vi "writeToXML.vi"(8 "error in (no error)":errorcluster, 10 "ClassLabel":string, 11 "CommandsForRotatorAxis in":refnum<class "CommandsForRotatorAxis.lvclass">) -> (0 "error out":errorcluster, 2 "XMLout":string, 3 "CommandsForRotatorAxis out":refnum<class "CommandsForRotatorAxis.lvclass">)   [LabVIEW 2014, in "TCSDataDefinitions.lvlib" / "TCSMountControlCommand.lvlib" / "CommandsForRotatorAxis.lvlib" / "CommandsForRotatorAxis.lvclass"]
uses:
  CommandsForRotatorAxis.lvclass
  TCSMCCCommand/TCSMCCCommand.lvclass
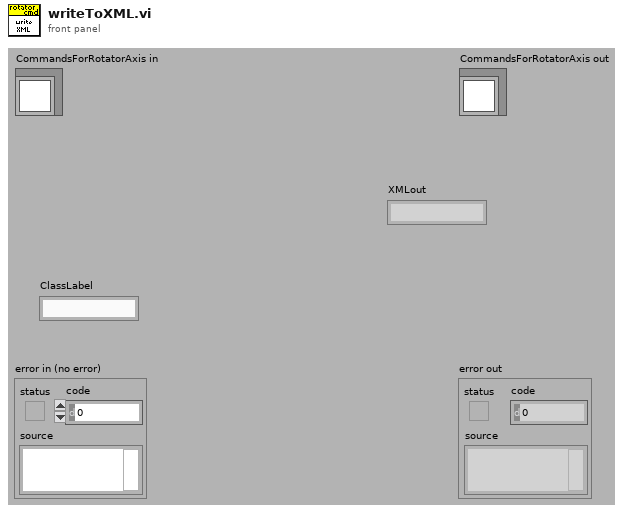
[diagram p1: front panel]
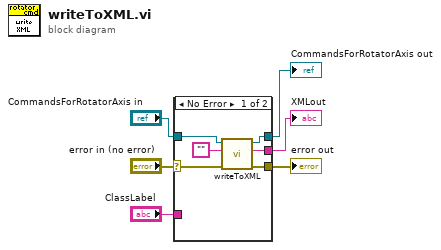
[diagram p0: block diagram]
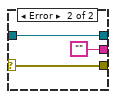
[diagram p2: hidden frame]
diagram:
  n1 = case shown="No Error" "error in (no error)" {
    selector: "error in (no error)" -> [w9 w15]
    tunnel: [w8 w15] -> w5
    tunnel: [w10 w14] -> w3
    tunnel: "CommandsForRotatorAxis in" -> [w12 w14]
    tunnel: [w7 ""] -> w2
    tunnel: "ClassLabel" -> [_ _]
    frame No Error {
      n2 = call-parent "writeToXML.vi"("error in (no error)"=w9, "ClassLabel"="", "TCSMCCCommand in"=w12) -> ("error out"=w8:errorcluster, "XMLout"=w7:string, "TCSMCCCommand out"=w10:refnum<class "CommandsForRotatorAxis.lvclass">)  [unwired: 6 in]
    }
    frame Error {
    }
  }
  "error out" <- w5
  "CommandsForRotatorAxis out" <- w3
  "XMLout" <- w2
